vi "ArrayOR.vi"(1 "Array 2":bool[](array[boolean]), 2 "Array 1":bool[](array[boolean])) -> (0 "1 || 2":bool[](array[boolean]))   [LabVIEW 2018]
panel:
  # "Array OR: ORs the two inputs together, outputting an array whose size\nis the size of the larger input array."
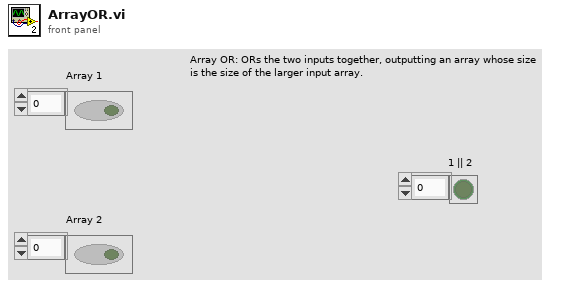
[diagram p1: front panel]
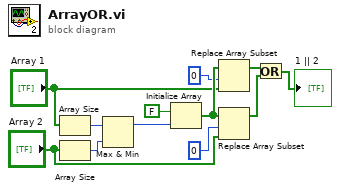
[diagram p0: block diagram]
diagram:
  n1 = Array Size(array="Array 1") -> (size(s)=w11:i32)
  n2 = Array Size(array="Array 2") -> (size(s)=w12:i32)
  n3 = Max & Min(x=w11, y=w12) -> (max(x,y)=w10:i32)  [unwired: 1 out]
  n4 = Initialize Array(FALSE, w10) -> (w8:bool[])
  n5 = Replace Array Subset(array=w8, new element="Array 1", index=0) -> (w2:bool[])
  n6 = Replace Array Subset(array=w8, new element="Array 2", index=0) -> (w3:bool[])
  n7 = Or(x=w2, y=w3) -> (x .or. y?=→"1 || 2":bool[])
